vi "set_enabled_state.vi"(8 "error in (no error)":errorcluster, 10 "haba":bool, 11 "ClockDL090202FPGA in":refnum<class "ClockDL090202FPGA.lvclass">) -> (0 "error out":errorcluster, 3 "ClockDL090202FPGA out":refnum<class "ClockDL090202FPGA.lvclass">)   [LabVIEW 2010, in "ClockDL090202FPGA.lvclass"]
uses:
  ClockDL090202FPGA.lvclass
  GenericClock/GenericClock/GenericClock.lvclass
  ClockDL090202FPGA.lvclass/ClockDL090202FPGA.ctl
  FPGAWrapper/GenericFPGAWrapper/GenericFPGAWrapper/GenericFPGAWrapper.lvclass
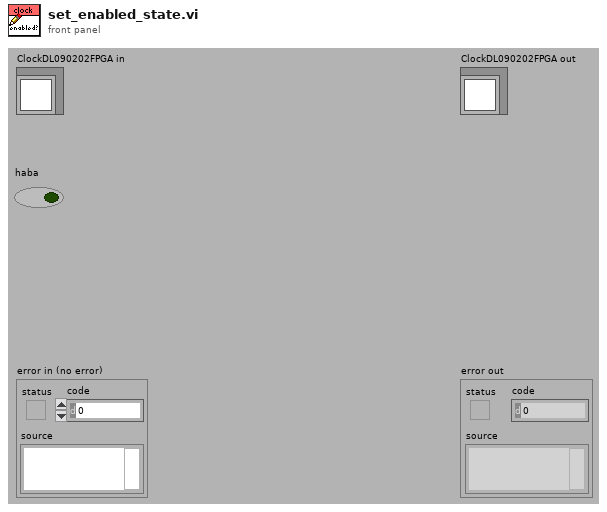
[diagram p1: front panel]
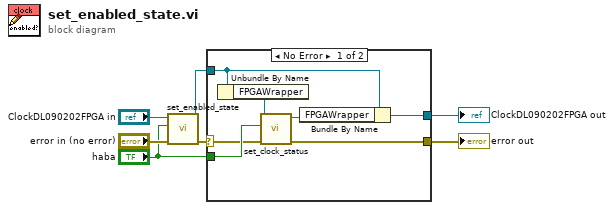
[diagram p0: block diagram]
diagram:
  n1 = call-parent "set_enabled_state.vi"("error in (no error)"="error in (no error)", "enabled?"="haba", "GenericClock in"="ClockDL090202FPGA in") -> ("error out"=w3:errorcluster, "GenericClock out"=w4:refnum<class "ClockDL090202FPGA.lvclass">)  [unwired: 7 in]
  n2 = case shown="No Error" w3 {
    selector: w3 -> [w12 w16]
    tunnel: "haba" -> [w13 _]
    tunnel: w4 -> [w9 w15]
    tunnel: [w11 w16] -> w2
    tunnel: [w8 w15] -> w1
    frame No Error {
      n3 = Unbundle By Name(w9) -> ("FPGAWrapper"=w14:refnum<class "GenericFPGAWrapper.lvclass">)
      n4 = call-dynamic "set_clock_status.vi"("error in (no error)"=w12, "enable clocks?"=w13, "GenericFPGAWrapper in"=w14) -> ("error out"=w11:errorcluster, "GenericFPGAWrapper out"=w10:refnum<class "GenericFPGAWrapper.lvclass">)  [unwired: 7 in]
      n5 = Bundle By Name(cluster=w9, "FPGAWrapper"=w10) -> (w8:refnum<class "ClockDL090202FPGA.lvclass">)
    }
    frame Error {
    }
  }
  "error out" <- w2
  "ClockDL090202FPGA out" <- w1
